vi "FP_Control Set Disable by Name.vi"(6 "FP Ctrl Properies":T1, 8 "Error":errorcluster, 11 "Control Label Array":string[](array[string])) -> (0 "Error Out":errorcluster, 3 "Success Out":bool)   [LabVIEW 2020]
uses:
  TypeDefs_Utility/ENUM_FP_Hide Show Disable.ctl
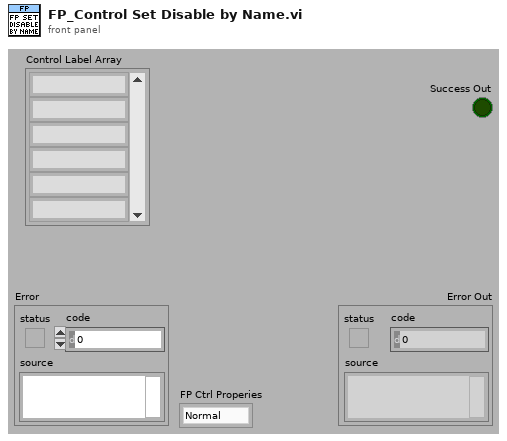
[diagram p1: front panel]
types:
  T1 = typedef "ENUM_FP_Hide Show Disable.ctl" = enum16{"Normal", "Disable", "Disable Gray", "Hide"}
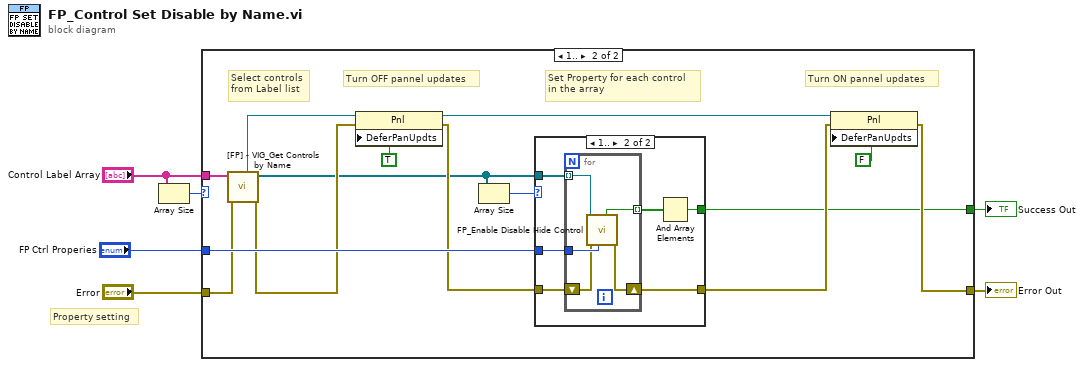
[diagram p0: block diagram]
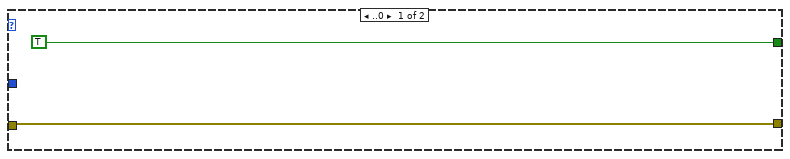
[diagram p2: hidden frame]
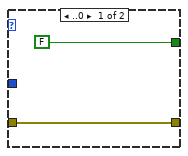
[diagram p3: hidden frame]
diagram:
  # "Property setting"
  n1 = Array Size(array="Control Label Array") -> (size(s)=w1:i32)
  n2 = case shown="1.." w1 {
    tunnel: "Error" -> [w7 w12]
    tunnel: "FP Ctrl Properies" -> [_ w18]
    tunnel: [TRUE w9] -> w4
    tunnel: "Control Label Array" -> [_ w15]
    tunnel: [w7 w20] -> w3
    frame ..0 {
    }
    frame 1.. {
      # "Set Property for each control\nin the array"
      # "Turn ON pannel updates"
      # "Turn OFF pannel updates"
      # "Select controls\nfrom Label list"
      n3 = call "[FP] - VIG_Get Controls by Name.vi"("Error"=w12, "Control Names"=w15) -> ("Error Out"=w13:errorcluster, "FP Controls Out"=w11:refnum<vi>[], "FrontPanel Out"=w14:refnum<vi>)  [unwired: 7 in]
      n4 = property class="Pnl"(reference=w14, error in=w13, "DeferPanUpdts"=TRUE ("Defer Panel Updates")) -> (reference out=w21:refnum<vi>, error out=w17:errorcluster)
      n5 = Array Size(array=w11) -> (size(s)=w10:i32)
      n6 = case shown="1.." w10 {
        tunnel: w18 -> [_ w30]
        tunnel: w17 -> [w24 w29]
        tunnel: [w24 w28] -> w16
        tunnel: [FALSE w25] -> w9
        tunnel: w11 -> [_ w27]
        frame ..0 {
        }
        frame 1.. {
          n7 = for {
            tunnel: w30 -> [w35]
            tunnel: w27 -> [w31] mode=indexing
            tunnel: [w32] -> w26 mode=indexing
            shift-right: [w34] -> w28
            shift-left: w29 -> [w33]
            n8 = call "FP_Enable Disable Hide Control.vi"("Settings"=w35, "Error"=w33, "Ctl Refnum"=w31) -> ("Error Out"=w34:errorcluster, "Success"=w32:bool)  [unwired: 4 in, 3 out]
          }
          n9 = And Array Elements(Boolean array=w26) -> (logical AND=w25:bool)
        }
      }
      n10 = property class="Pnl"(reference=w21, error in=w16, "DeferPanUpdts"=FALSE ("Defer Panel Updates")) -> (error out=w20:errorcluster)  [unwired: 1 out]
    }
  }
  "Success Out" <- w4
  "Error Out" <- w3
